vi "arm back.vi"   [LabVIEW 2020]
uses:
  Robot Global Data.vi
types:
  T1 = typedef "WPI_MotorControlDeviceRef.ctl" = cluster{"DeviceStatus":errorcluster, "Type":T2, "PWM":cluster{"PWM Channel":T3, "DeadBand":T4}, "CAN":cluster{"Device Number":u8, "SetOutput VI Ref":variant, "GetOutput VI Ref":variant, "Enable VI Ref":variant, "Disable VI Ref":variant, "Data":variant}, "Invert":bool, "DIO PWM":cluster{"PWM \"Enable\" Channel":T3, "DIOChannel":T5, "PWM Rate":dbl}}
  T2 = typedef "WPI_MotorControlType.ctl" = enum16{"PWM", "CAN", "DIO PWM"}
  T3 = typedef "FPGA_DIOPWMChannel.ctl" = enum8{"PWM 0", "PWM 1", "PWM 2", "PWM 3", "PWM 4", "PWM 5", "PWM 6", "PWM 7", "PWM 8", "PWM 9", "PWM MXP 0", "PWM MXP 1", "PWM MXP 2", "PWM MXP 3", "PWM MXP 4", "PWM MXP 5", "PWM MXP 6", "PWM MXP 7", "PWM MXP 8", "PWM MXP 9", "Invalid"}
  T4 = typedef "WPI_PWMDeadband.ctl" = cluster{"Name":string, "maxPositivePwm":i32, "minPositivePwm":i32, "centerPwm":i32, "maxNegativePwm":i32, "minNegativePwm":i32, "angularRange":u16}
  T5 = typedef "FPGA_DIOChannel.ctl" = enum8{"DIO 0", "DIO 1", "DIO 2", "DIO 3", "DIO 4", "DIO 5", "DIO 6", "DIO 7", "DIO 8", "DIO 9", "DIO MXP 0", "DIO MXP 1", "DIO MXP 2", "DIO MXP 3", "DIO MXP 4", "DIO MXP 5", "DIO MXP 6", "DIO MXP 7", "DIO MXP 8", "DIO MXP 9", "DIO MXP 10", "DIO MXP 11", "DIO MXP 12", "DIO MXP 13", "DIO MXP 14", "DIO MXP 15", "SPI Port CS1", "SPI Port CS2", "SPI Port CS3", "SPI Port MISO", "SPI Port MOSI", "Invalid"}
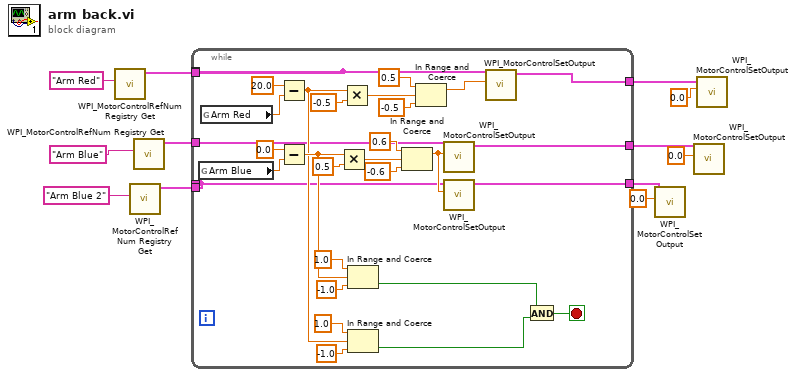
[diagram p0: block diagram]
diagram:
  n1 = call <vilib>:"WPI_MotorControlRefNum Registry Get.vi"("refnum name"="Arm Red") -> ("MotorControlDevRef"=w9:T1)  [unwired: 9 in, 1 out]
  n2 = call <vilib>:"WPI_MotorControlRefNum Registry Get.vi"("refnum name"="Arm Blue 2") -> ("MotorControlDevRef"=w7:T1)  [unwired: 9 in, 1 out]
  n3 = call <vilib>:"WPI_MotorControlRefNum Registry Get.vi"("refnum name"="Arm Blue") -> ("MotorControlDevRef"=w8:T1)  [unwired: 9 in, 1 out]
  n4 = while {
    tunnel: [w15] -> _
    tunnel: [w13] -> _
    tunnel: [w16] -> w5
    tunnel: [w18] -> w4
    tunnel: [w17] -> w6
    tunnel: w9 -> [w15]
    tunnel: w8 -> [w14]
    tunnel: w7 -> [w13]
    stop <- w41 stop-if-true
    n5 = global read "Robot Global Data.vi" "Arm Blue"() -> (w21:dbl)
    n6 = global read "Robot Global Data.vi" "Arm Red"() -> (w32:dbl)
    n7 = Subtract(x=20.0, y=w32) -> (x-y=w19:dbl)
    n8 = Subtract(x=0.0, y=w21) -> (x-y=w20:dbl)
    n9 = Multiply(x=w20, y=0.5) -> (x*y=w29:dbl)
    n10 = Multiply(x=w19, y=-0.5) -> (x*y=w28:dbl)
    n11 = In Range and Coerce(upper limit=1.0, x=w20, lower limit=-1.0) -> (In Range?=w40:bool)  [unwired: 1 out]
    n12 = In Range and Coerce(upper limit=1.0, x=w19, lower limit=-1.0) -> (In Range?=w39:bool)  [unwired: 1 out]
    n13 = In Range and Coerce(upper limit=0.6, x=w29, lower limit=-0.6) -> (coerced(x)=w24:dbl)  [unwired: 1 out]
    n14 = In Range and Coerce(upper limit=0.5, x=w28, lower limit=-0.5) -> (coerced(x)=w25:dbl)  [unwired: 1 out]
    n15 = call <vilib>:"WPI_MotorControlSetOutput.vi"("Output"=w24, "MotorControlDevRef"=w14) -> ("MotorControlDevRef"=w16:T1)  [unwired: 7 in, 2 out]
    n16 = call <vilib>:"WPI_MotorControlSetOutput.vi"("Output"=w24, "MotorControlDevRef"=w13) -> ("MotorControlDevRef"=w18:T1)  [unwired: 7 in, 2 out]
    n17 = call <vilib>:"WPI_MotorControlSetOutput.vi"("Output"=w25, "MotorControlDevRef"=w15) -> ("MotorControlDevRef"=w17:T1)  [unwired: 7 in, 2 out]
    n18 = And(x=w40, y=w39) -> (x .and. y?=w41:bool)
  }
  n19 = call <vilib>:"WPI_MotorControlSetOutput.vi"("Output"=0.0, "MotorControlDevRef"=w4) -> ()  [unwired: 7 in, 3 out]
  n20 = call <vilib>:"WPI_MotorControlSetOutput.vi"("Output"=0.0, "MotorControlDevRef"=w5) -> ()  [unwired: 7 in, 3 out]
  n21 = call <vilib>:"WPI_MotorControlSetOutput.vi"("Output"=0.0, "MotorControlDevRef"=w6) -> ()  [unwired: 7 in, 3 out]
